vi "Agilent_status.vi"(0 "VISA resource in":refnum<visa-resource-name>) -> (1 "VISA resource out":refnum<visa-resource-name>, 2 "Status string":string, 3 "Status Boolean":bool)   [LabVIEW 2017]
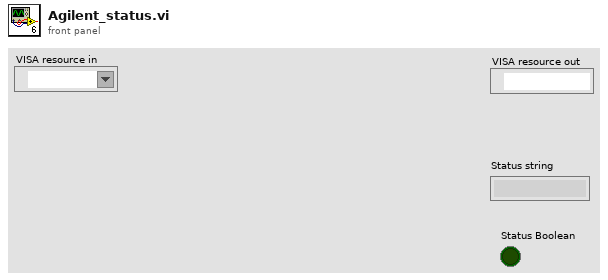
[diagram p1: front panel]
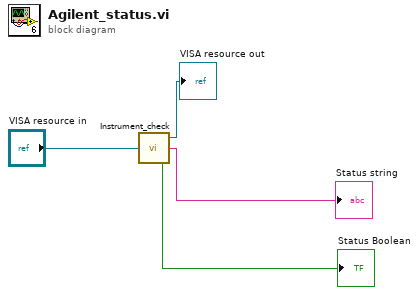
[diagram p0: block diagram]
diagram:
  n1 = call "Instrument_check.vi"("VISA resource in"="VISA resource in") -> ("VISA resource out"=→"VISA resource out":refnum<visa-resource-name>, "Response"=→"Status string":string, "Status"=→"Status Boolean":bool)
